vi "SetPoint.vi"(8 "error in (no error)":errorcluster, 10 "Point":refnum<class "Point.lvclass">, 11 "UMLClass in":refnum<class "UMLClass.lvclass">) -> (0 "error out":errorcluster, 3 "UMLClass out":refnum<class "UMLClass.lvclass">)   [LabVIEW 2021, in "Picture2D.lvlib" / "UMLClass.lvclass"]
uses:
  UMLClass.lvclass
  Shape/Shape.lvclass
  Point/Point.lvclass
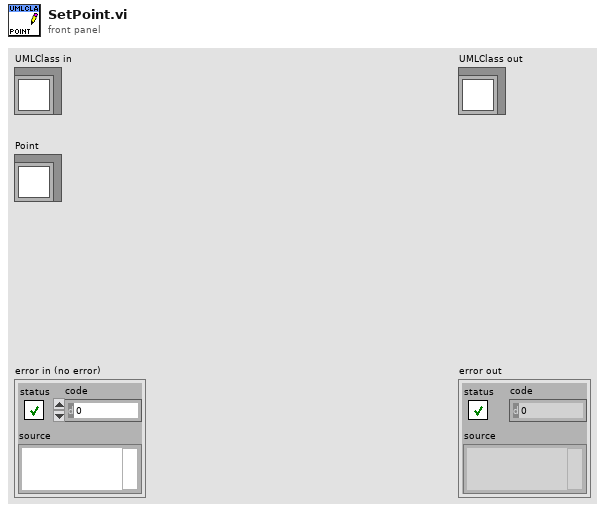
[diagram p1: front panel]
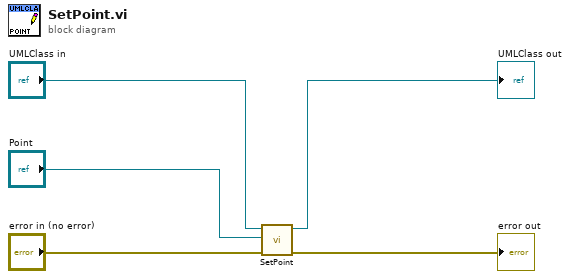
[diagram p0: block diagram]
diagram:
  n1 = call-parent "SetPoint.vi"("error in (no error)"="error in (no error)", "Point"="Point", "Picture2D in"="UMLClass in") -> ("error out"=→"error out":errorcluster, "Picture2D out"=→"UMLClass out":refnum<class "UMLClass.lvclass">)  [unwired: 7 in]
